vi "Community Initialize Resource.vi"(8 "error in (no error)":errorcluster, 11 "IConfiguration in":refnum<class "IConfiguration.lvclass">) -> (0 "error out":errorcluster, 3 "IConfiguration out":refnum<class "IConfiguration.lvclass">)   [LabVIEW 2017, in "Configuration.lvlib" / "IConfiguration.lvclass"]
uses:
  IConfiguration.lvclass
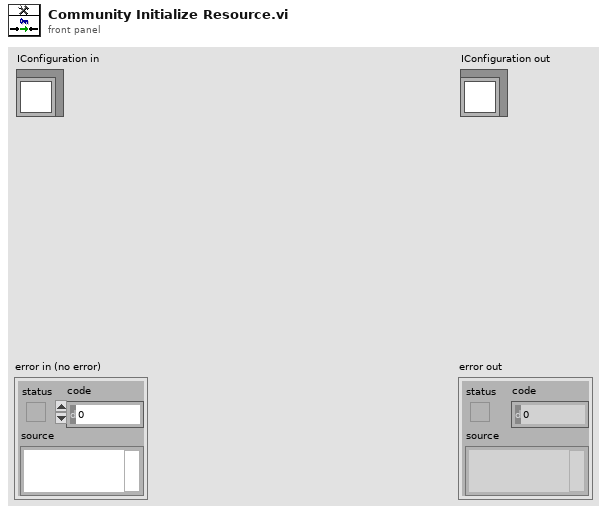
[diagram p1: front panel]
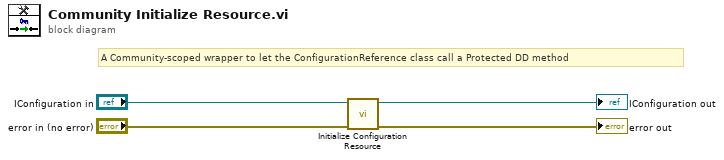
[diagram p0: block diagram]
diagram:
  # "A Community-scoped wrapper to let the ConfigurationReference class call a Protected DD method"
  n1 = call-dynamic "Initialize Configuration Resource.vi"("error in (no error)"="error in (no error)", "IConfiguration in"="IConfiguration in") -> ("error out"=→"error out":errorcluster, "IConfiguration out"=→"IConfiguration out":refnum<class "IConfiguration.lvclass">)  [unwired: 8 in]
